vi "SR830Monitor-new.vi"() -> ()   [LabVIEW 2016]
doc: "This VI is an example of storing and recovering data from the SR830 data buffers .\nDATA STORAGE RATE specifes the rate at which data is added to the data buffers .\nSCAN LENGTH specifies the approximate length of the data acquisition scan is seconds .\nPLOT GRAPH, PLOT CH 1 DATA and PLOT CH 2 DATA specify if the respective graphs will be displayed .\nAfter data storage is completed , the channel 1 and channel 2 points are downloaded from the instrument to the CH 1 POINTS and CH 2 POINTS arrays respectively . \nSince data recovered (using the SR830 receive message.vi) is in the string format , this VI requires a considerable amount of time to format the data into an array of floating point numbers . A quicker way would be to store the string in a file and use a CIN to speed up the process ."
uses:
  Utility/Monitor Communication/SR830/SR830-Cluster.ctl
  Global/Global Variables/Data_Display_global.vi
  Instrument_Setup.vi
panel:
  out "SR830":T1={"Lockin 1"=[], "X1"=0.0, "Y1"=0.0, "X1 Percent"=0.0, "X1 Overload"=FALSE, "Y1 Overload"=FALSE, "Unit X1"="nV", "Unit X2"="nV", "Unit X2a"="nV", "Unit X1a"="nV", "Sensitivity Setpoint"=26, "X1 Percent 2"=0.0} {"X1 Percent 2" scale=0.0..1.0; "Sensitivity Setpoint" items=["2 nV", "5 nV", "10 nV", "20 nV", "50 nV", "100 nV", "200 nV", "500 nV", "1 µV", "2 µV", "5 µV", "10 µV", "20 µV", "50 µV", "100 µV", "200 µV", "500 µV", "1 mV", "2 mV", "5 mV", "10 mV", "20 mV", "50 mV", "100 mV", "200 mV", "500 mV", "1 V", ""]; "X1 Percent" scale=0.0..1.0; "X1" format="%#4_5f"}
  out "AutoSet1":bool=TRUE
  in  "Stopp":bool
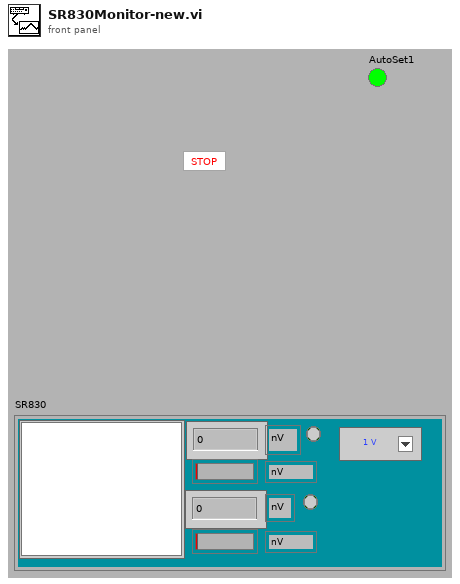
[diagram p1: front panel]
types:
  T1 = typedef "SR830-Cluster.ctl" = cluster{"Lockin 1":dbl[][], "X1":dbl, "Y1":dbl, "X1 Percent":dbl, "X1 Overload":bool, "Y1 Overload":bool, "Unit X1":string, "Unit X2":string, "Unit X2a":string, "Unit X1a":string, "Sensitivity Setpoint":i16, "X1 Percent 2":dbl}
  T2 = cluster{"error":bool, "code":i32, "source":string}
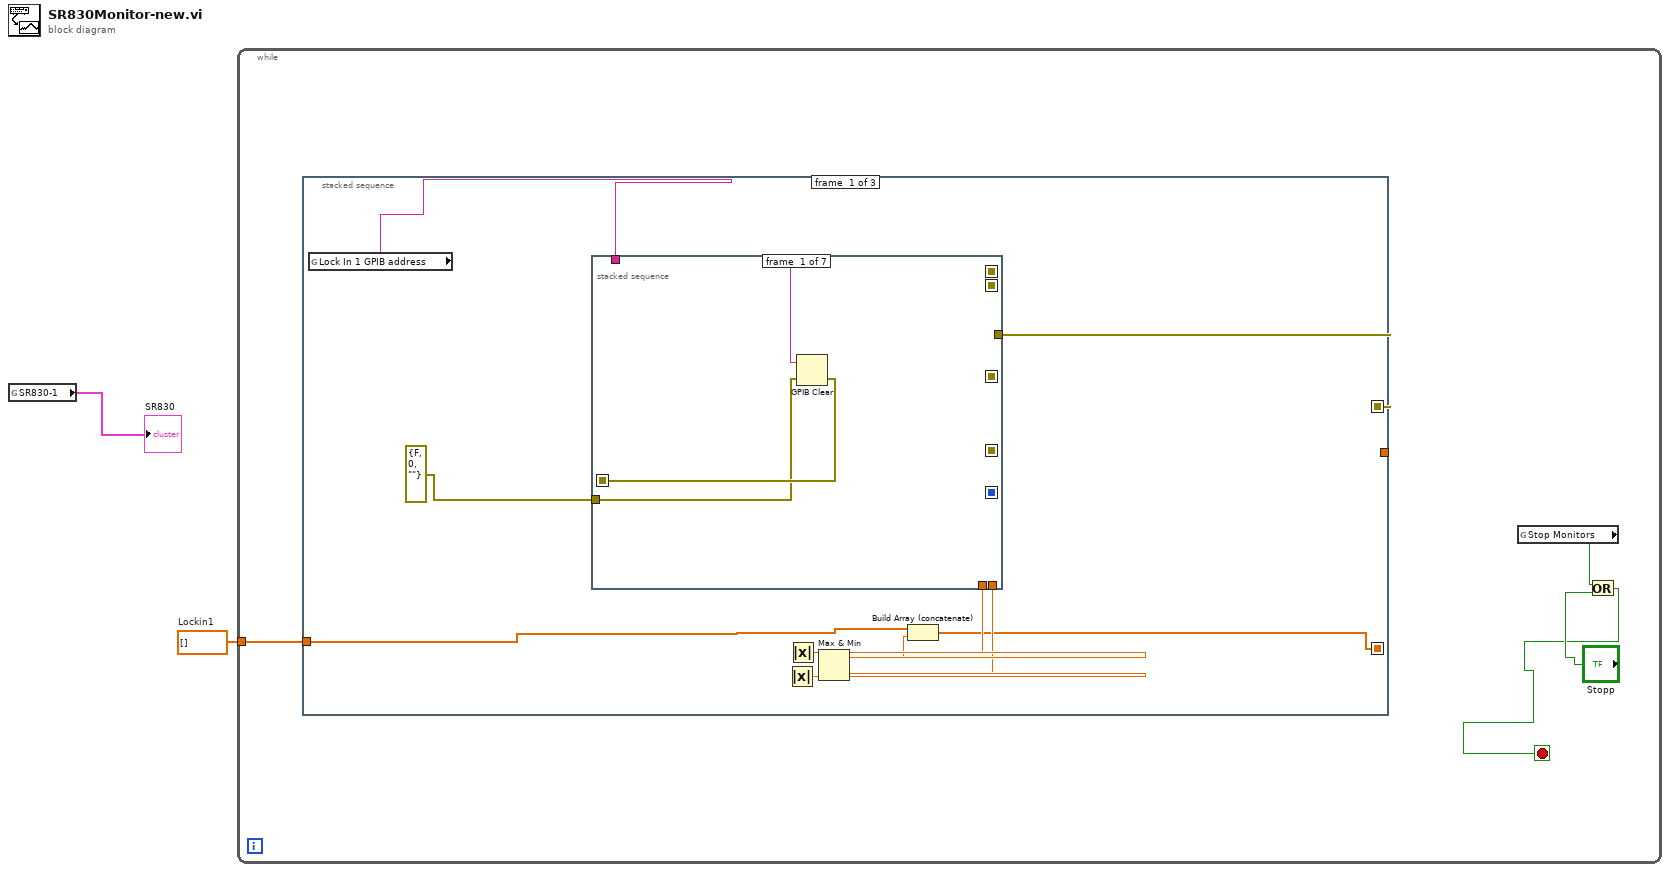
[diagram p0: block diagram]
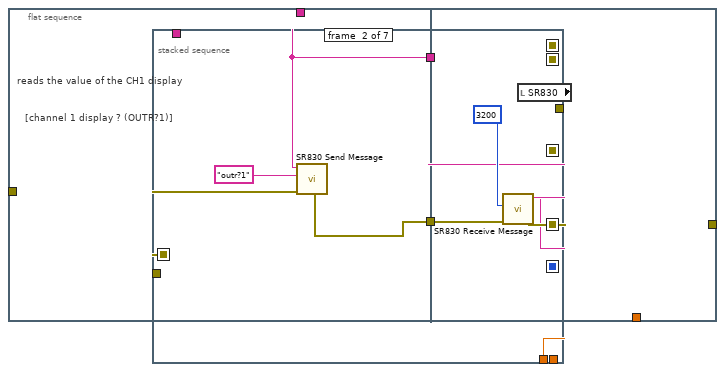
[diagram p2: hidden frame]
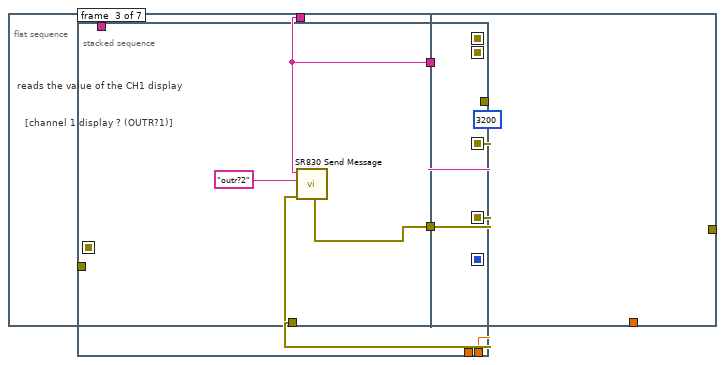
[diagram p3: hidden frame]
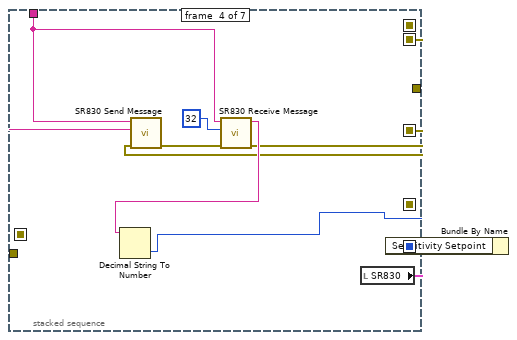
[diagram p4: hidden frame]
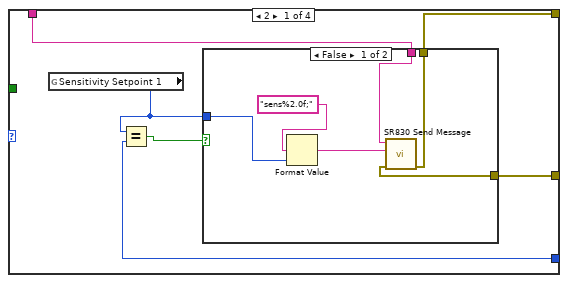
[diagram p6: hidden frame]
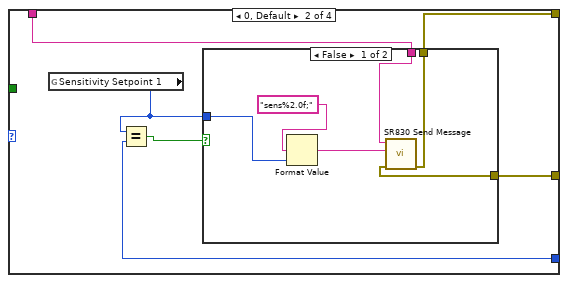
[diagram p8: hidden frame]
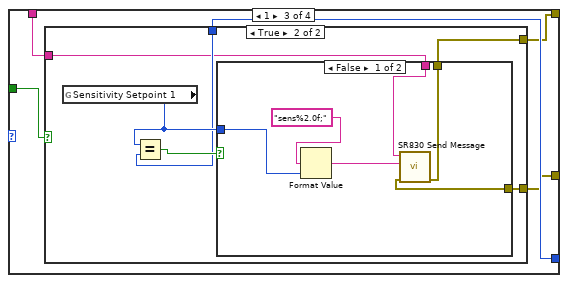
[diagram p10: hidden frame]
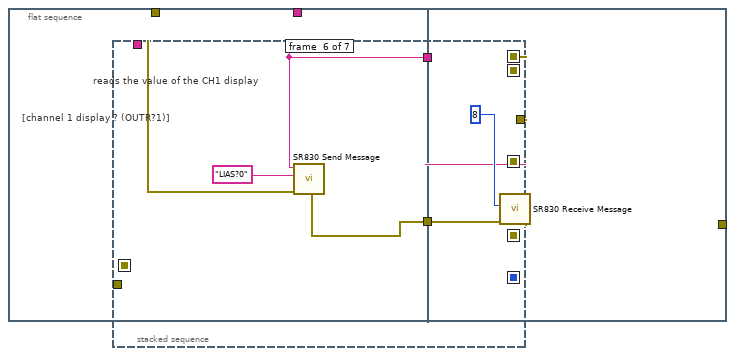
[diagram p13: hidden frame]
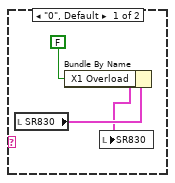
[diagram p14: hidden frame]
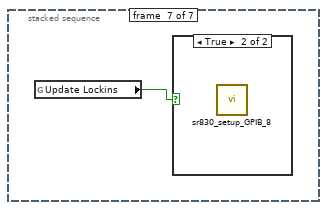
[diagram p15: hidden frame]
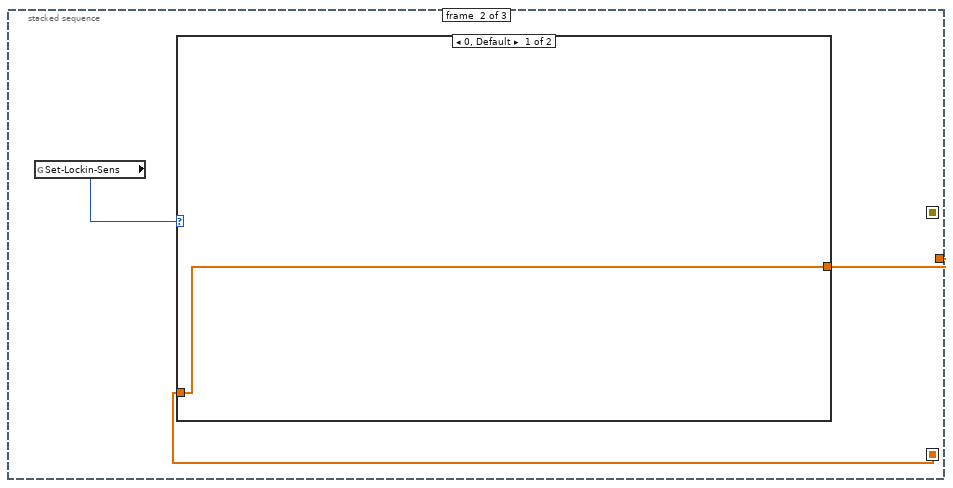
[diagram p17: hidden frame]
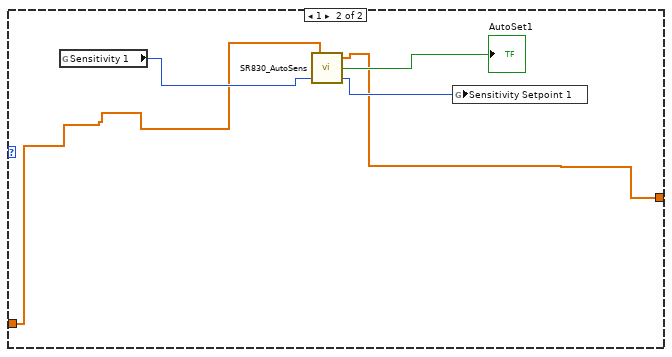
[diagram p18: hidden frame]
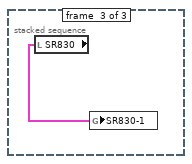
[diagram p19: hidden frame]
diagram:
  w1 = dbl[] []  # Lockin1
  n1 = global read "Data_Display_global.vi" "SR830-1"() -> (→"SR830":T1)
  n2 = while {
    tunnel: w1 -> [w3]
    stop <- w4 stop-if-true
    n3 = stacked-sequence {
      seq-local: [w16 _ _] -> [_ _ _]
      seq-local: [w7 _ _] -> [_ w139 _]
      tunnel: w3 -> [w8 _ _]
      tunnel: [_ w140 _] -> _
      frame #0 {
        n4 = global read "Instrument_Setup.vi" "Lock In 1 GPIB address"() -> (w10:string)
        n5 = stacked-sequence {
          seq-local: [_ w22 _ _ _ _ _] -> [_ _ w41 _ _ _ _]
          seq-local: [_ _ w39 _ _ _ _] -> [_ _ _ w60 _ _ _]
          seq-local: [w18 _ _ _ _ _ _] -> [_ w21 _ _ _ _ _]
          seq-local: [_ _ _ w59 _ _ _] -> [_ _ _ _ w71 _ _]
          seq-local: [_ _ _ w56 _ _ _] -> [_ _ _ _ w70 _ _]
          seq-local: [_ _ _ _ w68 _ _] -> [_ _ _ _ _ w118 _]
          tunnel: w10 -> [w19 w25 w40 w62 w69 w120 _]
          tunnel: [_ _ _ _ _ w119 _] -> w16
          tunnel: [_ w20 _ _ _ _ _] -> w13
          tunnel: [_ _ w38 _ _ _ _] -> w12
          tunnel: errorcluster {"status"=FALSE, "code"=0, "source"=""} ("error out") -> [w17 _ _ _ _ _ _]
          frame #0 {
            n6 = GPIB Clear(2:w17, 3:w19) -> (0:w18:errorcluster)  [unwired: 1 out]
          }
          frame #1 {
            n7 = flat-sequence {
              tunnel: w25 -> [w28]
              tunnel: [w28] -> w24
              tunnel: [w27] -> w23
              tunnel: w21 -> [w26]
              tunnel: w24 -> [w36]
              tunnel: w23 -> [w35]
              tunnel: [w34] -> w22
              tunnel: [w31] -> w20
              frame #0 {
                # "[channel 1 display ? (OUTR?1)]"
                # "reads the value of the CH1 display"
                n8 = call "SR830 Send Message.vi"("address string"=w28, "write buffer"="outr?1", "error in"=w26) -> ("error out"=w27:T2)  [unwired: 4 in, 2 out]
              }
              frame #1 {
                n9 = call "SR830 Receive Message.vi"("address string"=w36, "byte count"=3200, "error in"=w35) -> ("read buffer"=w33:string, "error out"=w34:T2)  [unwired: 4 in, 1 out]
                n10 = local read "SR830"() -> (w32:T1)
                n11 = Fract/Exp String To Number(string=w33) -> (number=w31:dbl)  [unwired: 3 in, 1 out]
                n12 = Bundle By Name(cluster=w32, "X1"=w31) -> (w30:T1)
                n13 = local write "SR830"(w30) -> ()
              }
            }
          }
          frame #2 {
            n14 = flat-sequence {
              tunnel: w40 -> [w46]
              tunnel: [w46] -> w43
              tunnel: [w45] -> w42
              tunnel: w41 -> [w44]
              tunnel: w43 -> [w54]
              tunnel: w42 -> [w53]
              tunnel: [w52] -> w39
              tunnel: [w48] -> w38
              frame #0 {
                # "[channel 1 display ? (OUTR?1)]"
                # "reads the value of the CH1 display"
                n15 = call "SR830 Send Message.vi"("address string"=w46, "write buffer"="outr?2", "error in"=w44) -> ("error out"=w45:T2)  [unwired: 4 in, 2 out]
              }
              frame #1 {
                n16 = call "SR830 Receive Message.vi"("address string"=w54, "byte count"=3200, "error in"=w53) -> ("read buffer"=w51:string, "error out"=w52:T2)  [unwired: 4 in, 1 out]
                n17 = local read "SR830"() -> (w50:T1)
                n18 = Fract/Exp String To Number(string=w51) -> (number=w48:dbl)  [unwired: 3 in, 1 out]
                n19 = Bundle By Name(cluster=w50, "Y1"=w48) -> (w49:T1)
                n20 = local write "SR830"(w49) -> ()
              }
            }
          }
          frame #3 {
            n21 = call "SR830 Send Message.vi"("address string"=w62, "write buffer"="sens?;", "error in"=w60) -> ("error out"=w64:T2)  [unwired: 4 in, 2 out]
            n22 = call "SR830 Receive Message.vi"("address string"=w62, "byte count"=32, "error in"=w64) -> ("read buffer"=w61:string, "error out"=w59:T2)  [unwired: 4 in, 1 out]
            n23 = Decimal String To Number(string=w61) -> (number=w56:i32)  [unwired: 2 in, 1 out]
            n24 = local read "SR830"() -> (w58:T1)
            n25 = Bundle By Name(cluster=w58, "Sensitivity Setpoint"=w56) -> (w57:T1)
            n26 = local write "SR830"(w57) -> ()
          }
          frame #4 {
            n27 = global read "Instrument_Setup.vi" "Set-Lockin-Sens"() -> (w67:u16)
            n28 = local read "AutoSet1"() -> (w66:bool)
            n29 = case shown="4" w67 {
              tunnel: w71 -> [w75 w88 w98 w117]
              tunnel: w70 -> [w74 w87 w101 _]
              tunnel: w69 -> [w73 w86 w100 _]
              tunnel: [w72 w85 w99 w117] -> w68
              tunnel: w66 -> [_ _ w102 _]
              frame 2 {
                n30 = global read "Data_Display_global.vi" "Sensitivity Setpoint 1"() -> (w76:i32)
                n31 = Equal?(x=w76, y=w74) -> (x = y?=w77:bool)
                n32 = case shown="False" w77 {
                  tunnel: w73 -> [w83 _]
                  tunnel: w76 -> [w82 _]
                  tunnel: w75 -> [w81 w84]
                  tunnel: [w80 w84] -> w72
                  frame False {
                    n33 = Format Value(format string="sens%2.0f;", value (0)=w82) -> (output string=w79:string)  [unwired: 1 in]
                    n34 = call "SR830 Send Message.vi"("address string"=w83, "write buffer"=w79, "error in"=w81) -> ("error out"=w80:T2)  [unwired: 4 in, 2 out]
                  }
                  frame True {
                  }
                }
              }
              frame 0, Default {
                n35 = global read "Data_Display_global.vi" "Sensitivity Setpoint 1"() -> (w89:i32)
                n36 = Equal?(x=w89, y=w87) -> (x = y?=w90:bool)
                n37 = case shown="False" w90 {
                  tunnel: w86 -> [w96 _]
                  tunnel: w89 -> [w95 _]
                  tunnel: w88 -> [w94 w97]
                  tunnel: [w93 w97] -> w85
                  frame False {
                    n38 = Format Value(format string="sens%2.0f;", value (0)=w95) -> (output string=w92:string)  [unwired: 1 in]
                    n39 = call "SR830 Send Message.vi"("address string"=w96, "write buffer"=w92, "error in"=w94) -> ("error out"=w93:T2)  [unwired: 4 in, 2 out]
                  }
                  frame True {
                  }
                }
              }
              frame 1 {
                n40 = case shown="True" w102 {
                  tunnel: w101 -> [_ w107]
                  tunnel: w100 -> [_ w106]
                  tunnel: [w103 w105] -> w99
                  tunnel: w98 -> [w103 w104]
                  frame False {
                  }
                  frame True {
                    n41 = global read "Data_Display_global.vi" "Sensitivity Setpoint 1"() -> (w108:i32)
                    n42 = Equal?(x=w108, y=w107) -> (x = y?=w109:bool)
                    n43 = case shown="False" w109 {
                      tunnel: w106 -> [w115 _]
                      tunnel: w108 -> [w114 _]
                      tunnel: w104 -> [w110 w116]
                      tunnel: [w113 w116] -> w105
                      frame False {
                        n44 = Format Value(format string="sens%2.0f;", value (0)=w114) -> (output string=w112:string)  [unwired: 1 in]
                        n45 = call "SR830 Send Message.vi"("address string"=w115, "write buffer"=w112, "error in"=w110) -> ("error out"=w113:T2)  [unwired: 4 in, 2 out]
                      }
                      frame True {
                      }
                    }
                  }
                }
              }
              frame 4 {
              }
            }
          }
          frame #5 {
            n46 = flat-sequence {
              tunnel: w120 -> [w125]
              tunnel: [w125] -> w122
              tunnel: [w124] -> w121
              tunnel: w118 -> [w123]
              tunnel: w122 -> [w130]
              tunnel: w121 -> [w129]
              tunnel: [w128] -> w119
              frame #0 {
                # "[channel 1 display ? (OUTR?1)]"
                # "reads the value of the CH1 display"
                n47 = call "SR830 Send Message.vi"("address string"=w125, "write buffer"="LIAS?0", "error in"=w123) -> ("error out"=w124:T2)  [unwired: 4 in, 2 out]
              }
              frame #1 {
                n48 = call "SR830 Receive Message.vi"("address string"=w130, "byte count"=8, "error in"=w129) -> ("read buffer"=w127:string, "error out"=w128:T2)  [unwired: 4 in, 1 out]
                n49 = case shown="\"1\"" w127 {
                  frame "0", Default {
                    n50 = local read "SR830"() -> (w134:T1)
                    n51 = Bundle By Name(cluster=w134, "X1 Overload"=FALSE) -> (w133:T1)
                    n52 = local write "SR830"(w133) -> ()
                  }
                  frame "1" {
                    n53 = local read "SR830"() -> (w137:T1)
                    n54 = Bundle By Name(cluster=w137, "Y1 Overload"=TRUE) -> (w136:T1)
                    n55 = local write "SR830"(w136) -> ()
                  }
                }
              }
            }
          }
          frame #6 {
            n56 = global read "Instrument_Setup.vi" "Update Lockins"() -> (w138:bool)
            n57 = case shown="True" w138 {
              frame False {
              }
              frame True {
                n58 = call "sr830_setup_GPIB_8.vi"() -> ()  [unwired: 3 in]
              }
            }
          }
        }
        n59 = Absolute Value(x=w12) -> (abs(x)=w14:dbl)
        n60 = Absolute Value(x=w13) -> (abs(x)=w15:dbl)
        n61 = Max & Min(x=w15, y=w14) -> (max(x,y)=w11:dbl)  [unwired: 1 out]
        n62 = Build Array (concatenate)(w8, w11) -> (w7:dbl[])
      }
      frame #1 {
        n63 = global read "Instrument_Setup.vi" "Set-Lockin-Sens"() -> (w141:u16)
        n64 = case shown="0, Default" w141 {
          tunnel: w139 -> [w142 w144]
          tunnel: [w142 w143] -> w140
          frame 0, Default {
          }
          frame 1 {
            n65 = global read "Data_Display_global.vi" "Sensitivity 1"() -> (w147:i32)
            n66 = call "SR830_AutoSens.vi"("Sensitivity"=w147, "Data in"=w144) -> ("Sensitivity Out"=w145:i32, "Set Sensitivity"=→"AutoSet1":bool, "Data out"=w143:dbl[])  [unwired: 1 in]
            n67 = global write "Data_Display_global.vi" "Sensitivity Setpoint 1"(w145) -> ()
          }
        }
      }
      frame #2 {
        n68 = local read "SR830"() -> (w148:T1)
        n69 = global write "Data_Display_global.vi" "SR830-1"(w148) -> ()
      }
    }
    n70 = global read "Data_Display_global.vi" "Stop Monitors"() -> (w6:bool)
    n71 = Or(x=w6, y="Stopp") -> (x .or. y?=w4:bool)
  }
